vi "WPI_ServoOpen.vi"(8 "error in (no error)":errorcluster, 9 "Angular Range":u16=170, 10 "PWM Channel":T2) -> (0 "error out":errorcluster, 3 "ServoDeviceRef":T1={"DeviceStatus"={"status"=FALSE, "code"=0, "source"=""}, "PWM Channel"=enum."Invalid", "DeadBand"={"Name"="", "maxPositivePwm"=0, "minPositivePwm"=0, "centerPwm"=0, "maxNegativePwm"=0, "minNegativePwm"=0, "angularRange"=0}})   [LabVIEW 2017]
doc: "Creates a reference to the servo controller you specify. You must open a reference before using any other VIs on this palette.\n\nThis software is licensed. Open the labview\\readme\\WPI Robotics Library Open Source License.txt file for more information."
uses:
  <vilib>/Rock Robotics/SystemInterfaces/DIO/FPGA_DIOPWMChannel.ctl
  <vilib>/Rock Robotics/WPI/PWM/Servo/WPI_ServoDeviceRef.ctl
  <vilib>/Rock Robotics/WPI/PWM/WPI_PWMDeadband.ctl
  <vilib>/Rock Robotics/WPI/PWM/WPI_PWMDeadband_ms.ctl
  <vilib>/Rock Robotics/WPI/PWM/WPI_PWMChannelCacheOp.ctl
  <vilib>/robotics/Simulator/Engine/ctl/DeviceID.ctl
  <vilib>/Rock Robotics/WPI/PWM/WPI_PWMPeriodMultiplier.ctl
  <vilib>/robotics/Simulator/NI_Robotics_Simulator.lvlib
  <instrlib>/Parallax Standard Servo/HAIOL/Simulator/Parallax Standard Servo Simulator.lvclass
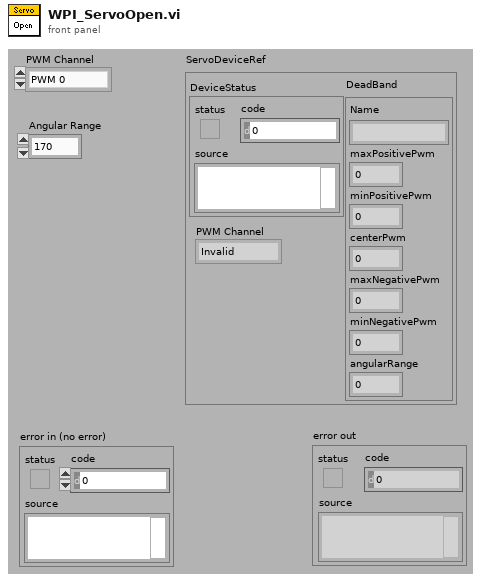
[diagram p1: front panel]
types:
  T1 = typedef "WPI_ServoDeviceRef.ctl" = cluster{"DeviceStatus":errorcluster, "PWM Channel":T2, "DeadBand":T3}
  T2 = typedef "FPGA_DIOPWMChannel.ctl" = enum8{"PWM 0", "PWM 1", "PWM 2", "PWM 3", "PWM 4", "PWM 5", "PWM 6", "PWM 7", "PWM 8", "PWM 9", "PWM MXP 0", "PWM MXP 1", "PWM MXP 2", "PWM MXP 3", "PWM MXP 4", "PWM MXP 5", "PWM MXP 6", "PWM MXP 7", "PWM MXP 8", "PWM MXP 9", "Invalid"}
  T3 = typedef "WPI_PWMDeadband.ctl" = cluster{"Name":string, "maxPositivePwm":i32, "minPositivePwm":i32, "centerPwm":i32, "maxNegativePwm":i32, "minNegativePwm":i32, "angularRange":u16}
  T4 = typedef "WPI_PWMDeadband_ms.ctl" = cluster{"Name":string, "maxPositivePwm":dbl, "minPositivePwm":dbl, "centerPwm":dbl, "maxNegativePwm":dbl, "minNegativePwm":dbl}
  T5 = typedef "NI_Robotics_Simulator.lvlib/DeviceID.ctl" = cluster{"robot ID":string, "sensor/actuator ID":string}
  T6 = typedef "WPI_PWMChannelCacheOp.ctl" = enum16{"Acquire", "Release", "Status"}
  T7 = typedef "WPI_PWMPeriodMultiplier.ctl" = u8
  T8 = typedef "WPI_DigitalModuleDeviceRef.ctl" = cluster{"DevStatus":errorcluster}
  T9 = typedef "WPI_PWMDeviceRef.ctl" = cluster{"DeviceStatus":errorcluster, "PWM Channel":T2}
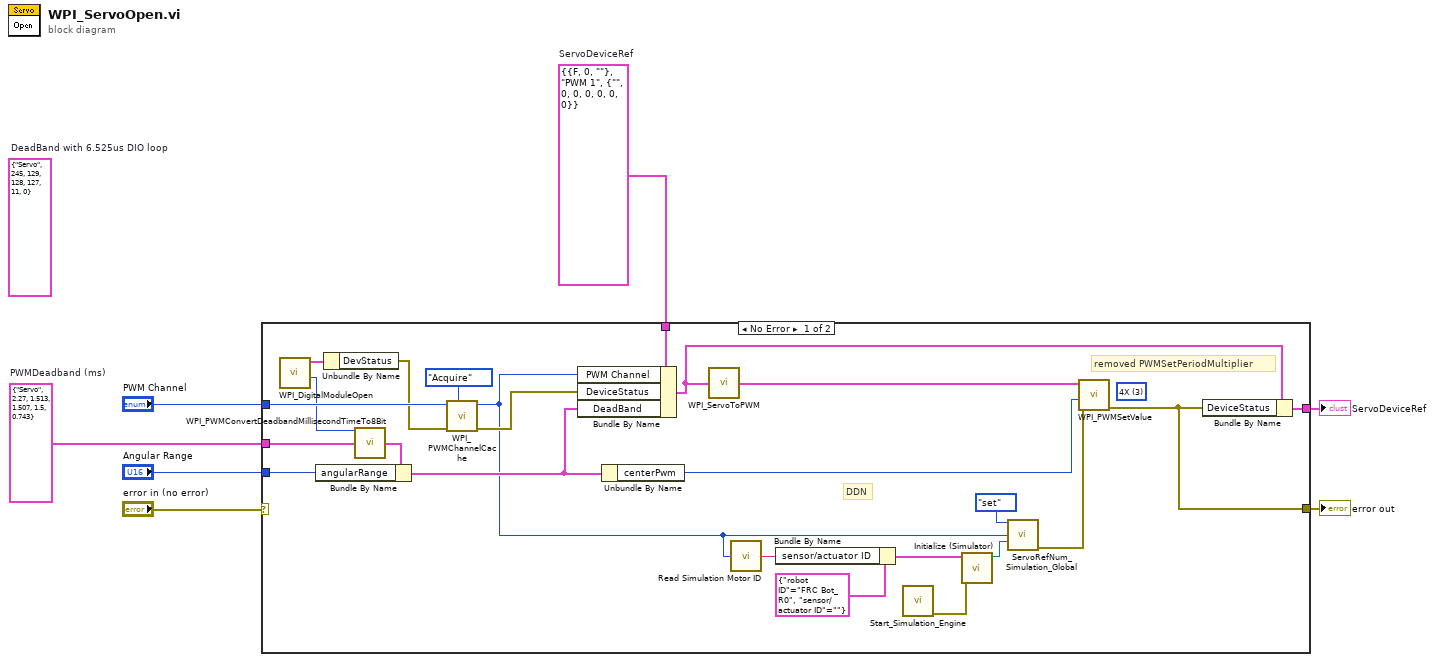
[diagram p0: block diagram]
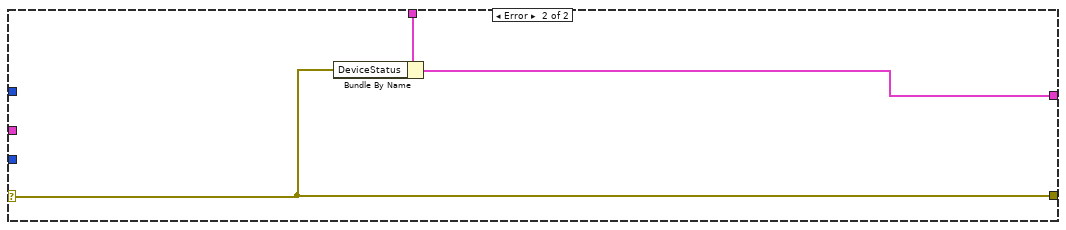
[diagram p2: hidden frame]
diagram:
  w1 = T4 {"Name"="Servo", "maxPositivePwm"=2.27, "minPositivePwm"=1.513, "centerPwm"=1.507, "maxNegativePwm"=1.5, "minNegativePwm"=0.743}  # PWMDeadband (ms)
  w5 = T1 {"DeviceStatus"={"status"=FALSE, "code"=0, "source"=""}, "PWM Channel"=enum."PWM 1", "DeadBand"={"Name"="", "maxPositivePwm"=0, "minPositivePwm"=0, "centerPwm"=0, "maxNegativePwm"=0, "minNegativePwm"=0, "angularRange"=0}}  # ServoDeviceRef
  (unwired) T3 {"Name"="Servo", "maxPositivePwm"=245, "minPositivePwm"=129, "centerPwm"=128, "maxNegativePwm"=127, "minNegativePwm"=11, "angularRange"=0}  # DeadBand with 6.525us DIO loop
  n1 = case shown="No Error" "error in (no error)" {
    selector: "error in (no error)" -> [_ w32]
    tunnel: "PWM Channel" -> [w28 _]
    tunnel: w5 -> [w30 w34]
    tunnel: [w22 w33] -> w6
    tunnel: [w8 w32] -> w7
    tunnel: "Angular Range" -> [w19 _]
    tunnel: w1 -> [w18 _]
    frame No Error {
      (unwired) T7 3 items=["1X"=0, "2X"=1, "4X"=3] ("PWMPeriodMultiplier")
      # "removed PWMSetPeriodMultiplier"
      # "DDN"
      n2 = call <vilib>:"WPI_DigitalModuleOpen.vi"() -> ("LoopTiming"=w17:u16, "DigitalModuleDevRef"=w27:T8)  [unwired: 2 in, 8 out]
      n3 = Unbundle By Name(w27) -> ("DevStatus"=w26:errorcluster)
      n4 = call <vilib>:"WPI_PWMConvertDeadbandMillisecondTimeTo8Bit.vi"("DIO Loop Timing (ticks)"=w17, "PWMDeadband (ms)"=w18) -> ("PWMDeadband Coefficient"=w21:T3)  [unwired: 13 in]
      n5 = Bundle By Name(cluster=w21, "angularRange"=w19) -> (w20:T3)
      n6 = call <vilib>:"WPI_PWMChannelCache.vi"("Operation"=WPI_PWMChannelCacheOp."Acquire", "error in (no error)"=w26, "PWMChannel"=w28) -> ("error out"=w29:errorcluster, "AllocatedPWMChannel"=w10:T2)  [unwired: 2 in, 5 out]
      n7 = Bundle By Name(cluster=w30, "PWM Channel"=w10, "DeviceStatus"=w29, "DeadBand"=w20) -> (w23:T1)
      n8 = Unbundle By Name(w20) -> ("centerPwm"=w25:i32)
      n9 = call <vilib>:"WPI_ServoToPWM.vi"("ServoDeviceRef"=w23) -> ("PWMDeviceRef"=w24:T9)
      n10 = call <vilib>:"Read Simulation Motor ID.vi"("PWM.PWM Channel"=w10) -> ("motor ID"=w12:string)  [unwired: 13 in, 1 out]
      n11 = Bundle By Name(cluster=T5 {"robot ID"="FRC Bot_R0", "sensor/actuator ID"=""} ("Device ID"), "sensor/actuator ID"=w12) -> (w13:T5)
      n12 = call <vilib>:"Start_Simulation_Engine.vi"() -> ("error out"=w14:errorcluster)  [unwired: 15 in]
      n13 = call <instrlib>:"Initialize (Simulator).vi"("error in (no error)"=w14, "Device ID"=w13) -> ("Parallax Standard Servo out"=w15:refnum<class "Parallax Standard Servo.lvclass">)  [unwired: 8 in, 1 out]
      n14 = call <vilib>:"ServoRefNum_Simulation_Global.vi"("menu"=enum16{"set", "get", "delete"}."set", "PWM Channel"=w10, "Servo Set"=w15) -> ("error out"=w9:errorcluster)  [unwired: 11 in, 1 out]
      n15 = call <vilib>:"WPI_PWMSetValue.vi"("error in (no error)"=w9, "Value"=w25, "PWMDeviceRef"=w24) -> ("error out"=w8:errorcluster)  [unwired: 1 in, 7 out]
      n16 = Bundle By Name(cluster=w23, "DeviceStatus"=w8) -> (w22:T1)
    }
    frame Error {
      n17 = Bundle By Name(cluster=w34, "DeviceStatus"=w32) -> (w33:T1)
    }
  }
  "ServoDeviceRef" <- w6
  "error out" <- w7
